vi "CH_LM get Communication Mode.vi"(2 "error in (no error)":errorcluster) -> (0 "error out":errorcluster, 1 "Communication Mode":T1=enum."USB")   [LabVIEW 2012, in "CH_LM.lvlib"]
doc: "This VI returns the communictation mode."
uses:
  CH_LM.lvlib
  CH_LM Communication Mode.ctl
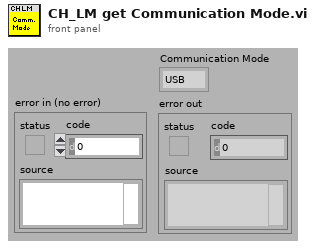
[diagram p1: front panel]
types:
  T1 = typedef "CH_LM.lvlib/CH_LM Communication Mode.ctl" = enum16{"None", "USB", "GPIB", "RS232"}
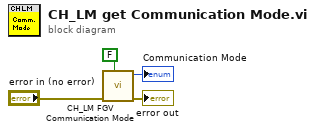
[diagram p0: block diagram]
diagram:
  n1 = call "CH_LM FGV Communication Mode.vi"("set? (False)"=FALSE, "error in (no error)"="error in (no error)") -> ("error out"=→"error out":errorcluster, "Communication Mode"=→"Communication Mode":T1)  [unwired: 1 in, 4 out]
